vi "SelectData.vi"(8 "error in (no error)":errorcluster, 11 "DataBase in":refnum<class "DataBase.lvclass">) -> (0 "error out":errorcluster, 3 "DataBase out":refnum<class "DataBase.lvclass">)   [LabVIEW 2019, in "DataBase.lvlib" / "DataBase.lvclass"]
uses:
  DataBase.lvclass
  DataBase.lvclass/DataBase.ctl
  <vilib>/addons/database/_DB Variant To Data/Database Variant To Data.xnode
  <vilib>/addons/database/NI_Database_API.lvlib
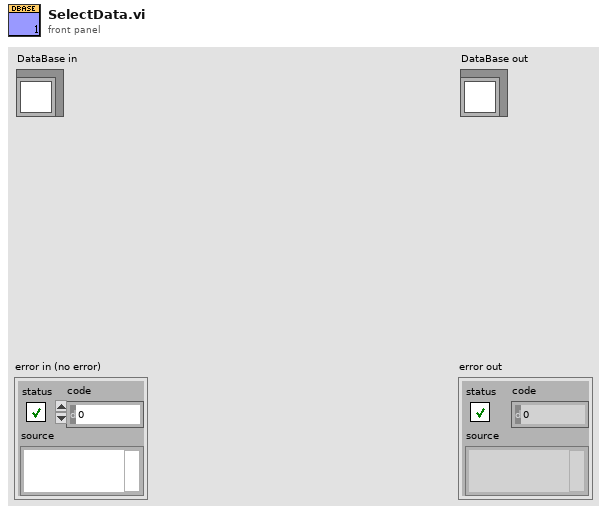
[diagram p1: front panel]
types:
  T1 = typedef "NI_Database_API.lvlib/Conn ObjectReference.ctl" = refnum<k1>
  T2 = enum16{"Station 1", "Station 2", "Station 3", "Station 4"}
  T3 = enum16{"OneDay", "OneWeek", "OneMonth", "OneYear"}
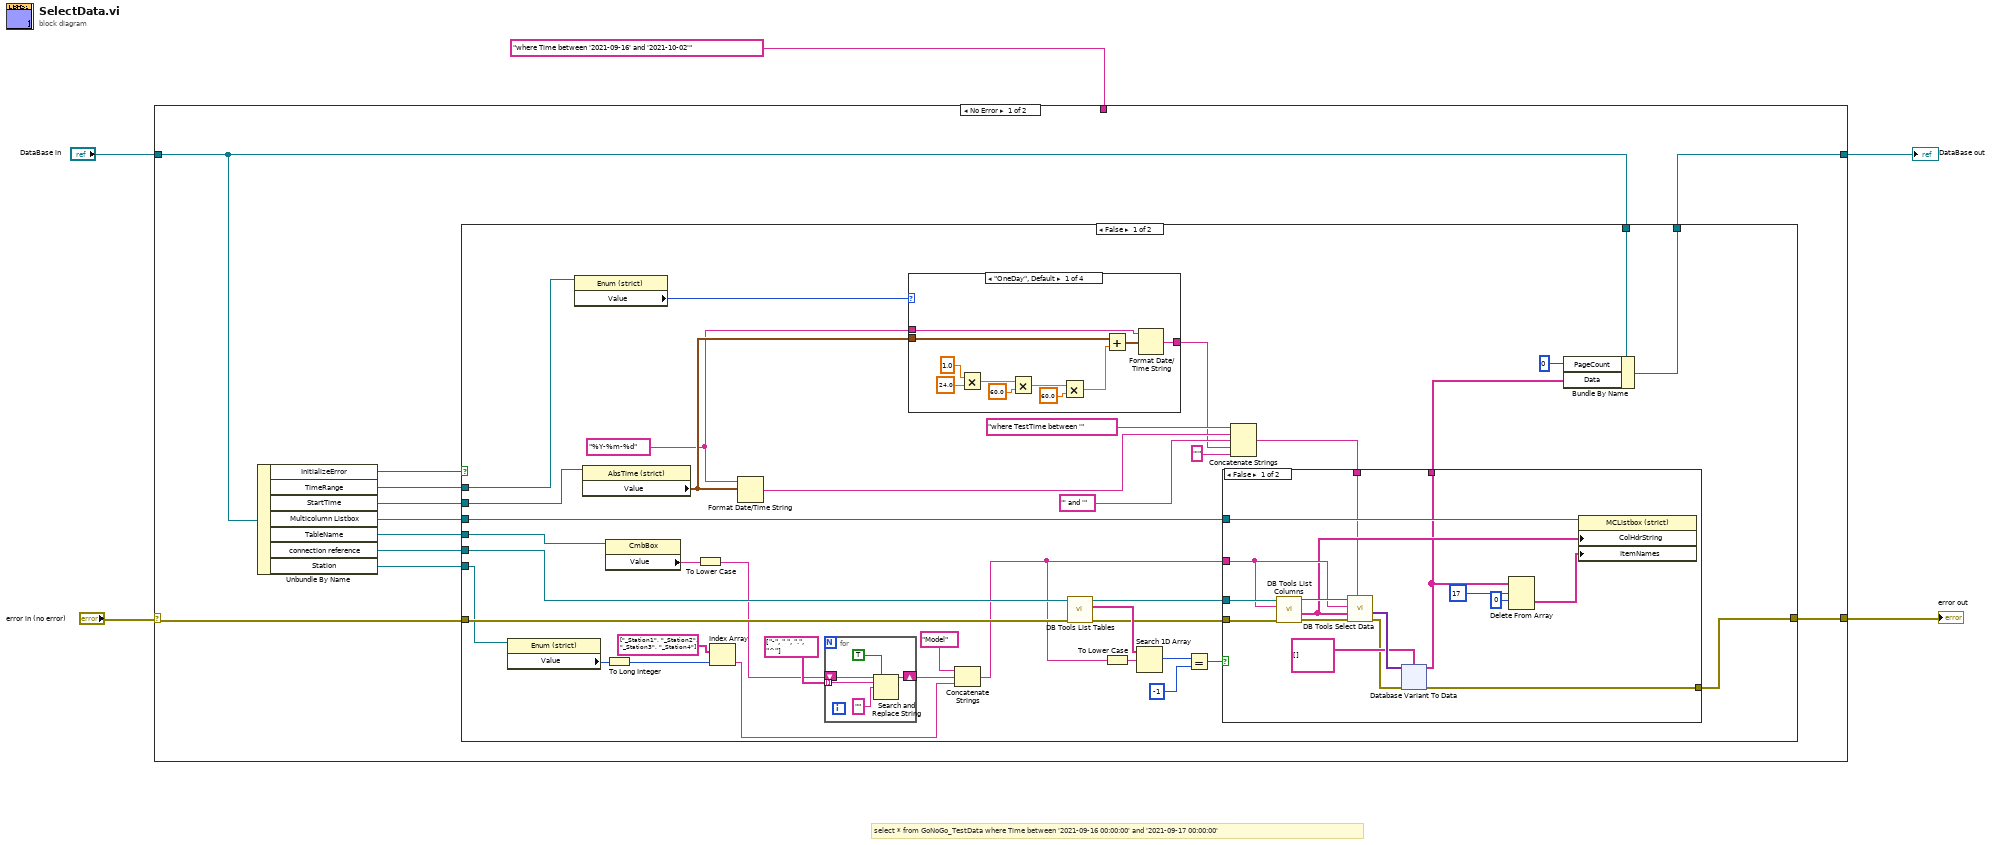
[diagram p0: block diagram]
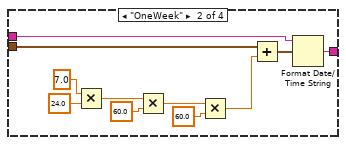
[diagram p2: hidden frame]
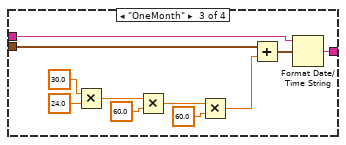
[diagram p3: hidden frame]
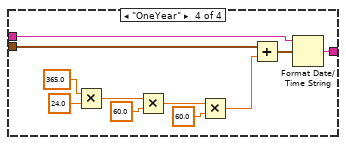
[diagram p4: hidden frame]
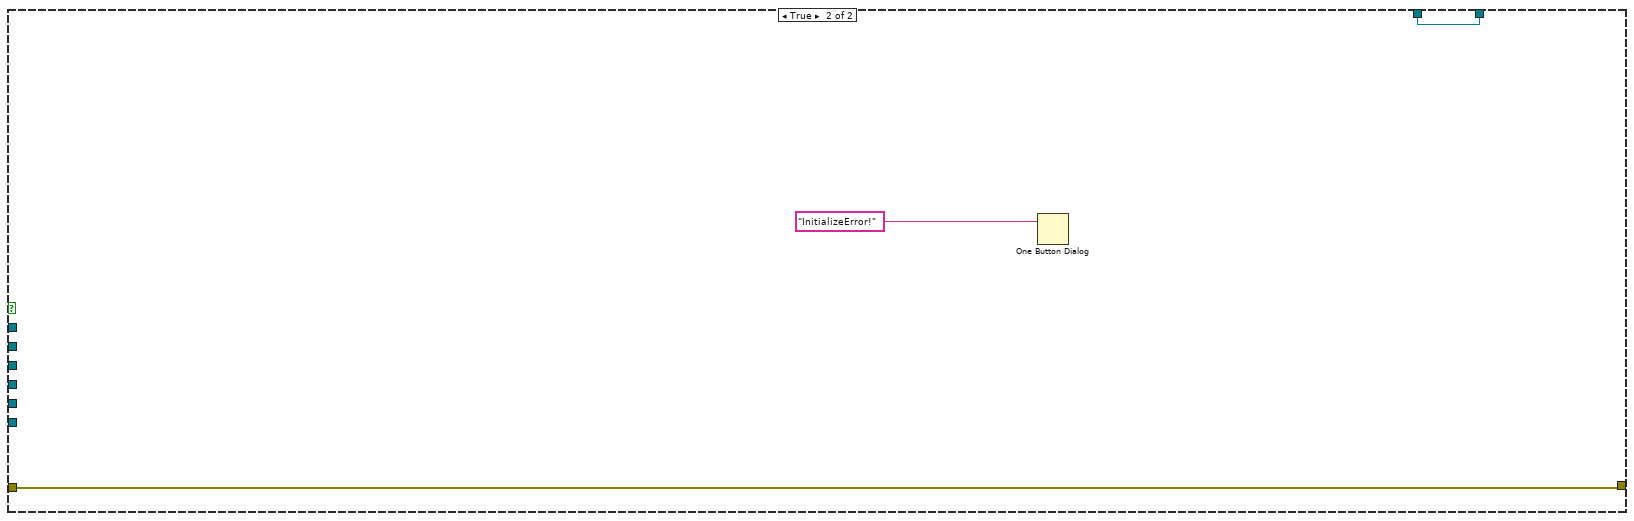
[diagram p6: hidden frame]
diagram:
  # "select * from GoNoGo_TestData where Time between '2021-09-16 00:00:00' and '2021-09-17 00:00:00'"
  n1 = case shown="No Error" "error in (no error)" {
    selector: "error in (no error)" -> [w14 w169]
    tunnel: [w13 w169] -> w4
    tunnel: [w9 w168] -> w2
    tunnel: "DataBase in" -> [w10 w168]
    tunnel: "where Time between '2021-09-16' and '2021-10-02'" ("condition") -> [_ _]
    frame No Error {
      n2 = Unbundle By Name(w10) -> ("InitializeError"=w7:bool, "TimeRange"=w11:refnum<vi>, "StartTime"=w12:refnum<vi>, "Multicolumn Listbox"=w16:refnum<vi>, "TableName"=w8:refnum<vi>, "connection reference"=w15:T1, "Station"=w6:refnum<vi>)
      n3 = case shown="False" w7 {
        tunnel: w16 -> [w47 _]
        tunnel: w15 -> [w46 _]
        tunnel: w14 -> [w45 w166]
        tunnel: [w44 w166] -> w13
        tunnel: w12 -> [w43 _]
        tunnel: w11 -> [w40 _]
        tunnel: w10 -> [w32 w167]
        tunnel: [w29 w167] -> w9
        tunnel: w8 -> [w27 _]
        tunnel: w6 -> [w21 _]
        frame False {
          w33 = "%Y-%m-%d" ("time format string (%c)")
          n4 = property class="Enum (strict)"(reference=w21) -> ("Value"=w18:T2)  [unwired: 1 in, 2 out]
          n5 = property class="Enum (strict)"(reference=w40) -> ("Value"=w34:T3)  [unwired: 1 in, 2 out]
          n6 = property class="AbsTime (strict)"(reference=w43) -> ("Value"=w35:timestamp)  [unwired: 1 in, 2 out]
          n7 = property class="CmbBox"(reference=w27) -> ("Value"=w28:string)  [unwired: 1 in, 2 out]
          n8 = To Long Integer(number=w18) -> (32bit integer=w20:i32)
          n9 = To Lower Case(string=w28) -> (all lower case string=w25:string)
          n10 = Index Array(array=string[] ["_Station1", "_Station2", "_Station3", "_Station4"], index=w20) -> (element=w17:string)
          n11 = Format Date/Time String(time format string (%c)=w33, seconds (now)=w35) -> (date/time string=w39:string)  [unwired: 1 in]
          n12 = for {
            tunnel: string[] ["-", " ", ".", "^"] -> [w59] mode=indexing
            shift-right: [w56] -> w24
            shift-left: w25 -> [w57]
            n13 = Search and Replace String(replace all?=TRUE ("replace all? (F)"), input string=w57, search string=w59, replace string="" ("replace string (\"\")")) -> (result string=w56:string)  [unwired: 4 in, 3 out]
          }
          n14 = case shown="\"OneDay\", Default" w34 {
            tunnel: [w60 w71 w82 w93] -> w38
            tunnel: w35 -> [w64 w72 w83 w94]
            tunnel: w33 -> [w61 w73 w84 w95]
            frame "OneDay", Default {
              n15 = Multiply(x=1.0, y=24.0) -> (x*y=w66:dbl)
              n16 = Multiply(x=w66, y=60.0) -> (x*y=w69:dbl)
              n17 = Multiply(x=w69, y=60.0) -> (x*y=w63:dbl)
              n18 = Add(x=w64, y=w63) -> (x+y=w62:timestamp)
              n19 = Format Date/Time String(time format string (%c)=w61, seconds (now)=w62) -> (date/time string=w60:string)  [unwired: 1 in]
            }
            frame "OneWeek" {
              n20 = Multiply(x=7.0, y=24.0) -> (x*y=w77:dbl)
              n21 = Multiply(x=w77, y=60.0) -> (x*y=w80:dbl)
              n22 = Multiply(x=w80, y=60.0) -> (x*y=w75:dbl)
              n23 = Add(x=w72, y=w75) -> (x+y=w74:timestamp)
              n24 = Format Date/Time String(time format string (%c)=w73, seconds (now)=w74) -> (date/time string=w71:string)  [unwired: 1 in]
            }
            frame "OneMonth" {
              n25 = Multiply(x=30.0, y=24.0) -> (x*y=w88:dbl)
              n26 = Multiply(x=w88, y=60.0) -> (x*y=w91:dbl)
              n27 = Multiply(x=w91, y=60.0) -> (x*y=w86:dbl)
              n28 = Add(x=w83, y=w86) -> (x+y=w85:timestamp)
              n29 = Format Date/Time String(time format string (%c)=w84, seconds (now)=w85) -> (date/time string=w82:string)  [unwired: 1 in]
            }
            frame "OneYear" {
              n30 = Multiply(x=365.0, y=24.0) -> (x*y=w99:dbl)
              n31 = Multiply(x=w99, y=60.0) -> (x*y=w102:dbl)
              n32 = Multiply(x=w102, y=60.0) -> (x*y=w97:dbl)
              n33 = Add(x=w94, y=w97) -> (x+y=w96:timestamp)
              n34 = Format Date/Time String(time format string (%c)=w95, seconds (now)=w96) -> (date/time string=w93:string)  [unwired: 1 in]
            }
          }
          n35 = Concatenate Strings("Model" ("string"), w24, w17) -> (w23:string)
          n36 = call <vilib>:"DB Tools List Tables.vi"("error in (no error)"=w45, "connection reference"=w46) -> ("error out"=w50:errorcluster, "tables"=w54:string[], "connection reference out"=w48:T1)  [unwired: 3 in]
          n37 = To Lower Case(string=w23) -> (all lower case string=w51:string)
          n38 = Search 1D Array(1D array=w54, element=w51) -> (index of element=w53:i32)  [unwired: 1 in]
          n39 = Equal?(x=w53, y=-1) -> (x = y?=w49:bool)
          n40 = Concatenate Strings("where TestTime between '" ("condition"), w39, "' and '" ("string"), w38, "'" ("string")) -> (w36:string)
          n41 = case shown="False" w49 {
            tunnel: w50 -> [w118 w164]
            tunnel: w48 -> [w119 _]
            tunnel: w23 -> [w115 _]
            tunnel: w47 -> [w117 _]
            tunnel: [w109 w164] -> w44
            tunnel: w36 -> [w108 _]
            tunnel: [w107 _] -> w31
            frame False {
              n42 = call <vilib>:"DB Tools List Columns.vi"("error in (no error)"=w118, "table"=w115, "connection reference"=w119) -> ("error out"=w113:errorcluster, "columns"=w114:string[], "connection reference out"=w116:T1)  [unwired: 1 in, 1 out]
              n43 = call <vilib>:"DB Tools Select Data.vi"("condition"=w108, "error in (no error)"=w113, "columns"=w114, "table"=w115, "connection reference"=w116) -> ("error out"=w110:errorcluster, "data"=w112:variant[][])  [unwired: 1 in, 1 out]
              n44 = xnode "Database Variant To Data"("database variant"=w112, "error in (no error)"=w110, "type"=string[][] []) -> ("data"=w107:string[][], "error out"=w109:errorcluster)
              n45 = Delete From Array(array=w107, length=17, index (row)=0) -> (deleted portion=w105:string[][])  [unwired: 1 in, 1 out]
              n46 = property class="MCListbox (strict)"(reference=w117, "ColHdrString"=w114, "ItemNames"=w105) -> ()  [unwired: 1 in, 2 out]
            }
            frame True {
            }
          }
          n47 = Bundle By Name(cluster=w32, "PageCount"=0, "Data"=w31) -> (w29:refnum<class "DataBase.lvclass">)
        }
        frame True {
          n48 = One Button Dialog(message="InitializeError!") -> ()  [unwired: 1 in, 1 out]
        }
      }
    }
    frame Error {
    }
  }
  "error out" <- w4
  "DataBase out" <- w2
